vi "SR830-ENBW-WaitTime-Tau-FilterSlope.vi"(8 "error in (no error)":errorcluster, 11 "VISA resource name":refnum<visa-resource-name>) -> (0 "error out":errorcluster, 3 "VISA resource name out":refnum<visa-resource-name>, 4 "Wait Time (s)":dbl, 5 "Filter slope (dB/oct)":dbl, 6 "ENBW":dbl, 7 "Time Constant (s)":dbl)   [LabVIEW 2016]
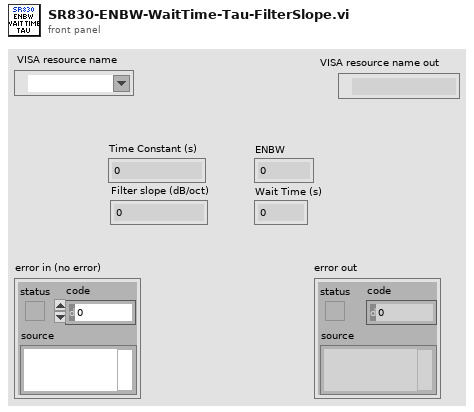
[diagram p1: front panel]
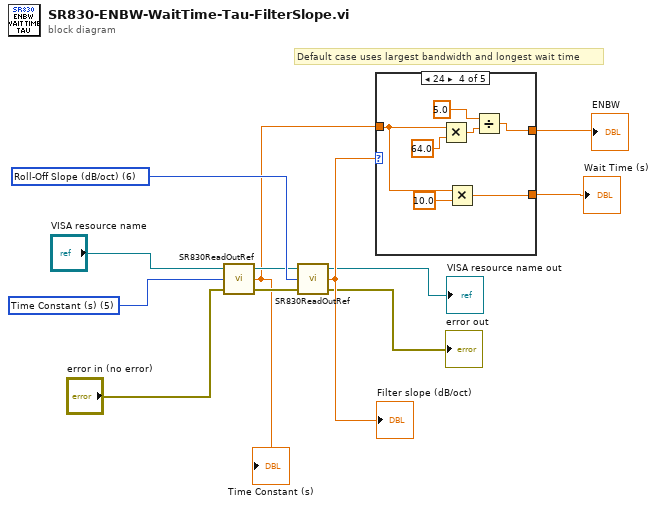
[diagram p0: block diagram]
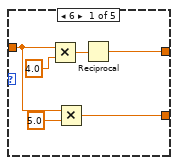
[diagram p2: hidden frame]
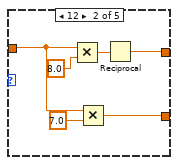
[diagram p3: hidden frame]
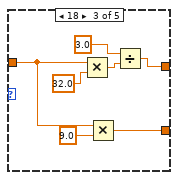
[diagram p4: hidden frame]
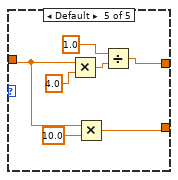
[diagram p5: hidden frame]
diagram:
  w9 = u16 6 items=["Voltage Out (Vrms)"=1, "Frequency (Hz)"=2, "Aux Out 1 (VDC)"=3, "Aux Out 2 (VDC)"=4, "Time Constant (s)"=5, "Roll-Off Slope (dB/oct)"=6] ("ReadOut (1: Voltage Amplitude)")
  w10 = u16 5 items=["Voltage Out (Vrms)"=1, "Frequency (Hz)"=2, "Aux Out 1 (VDC)"=3, "Aux Out 2 (VDC)"=4, "Time Constant (s)"=5, "Roll-Off Slope (dB/oct)"=6] ("ReadOut (1: Voltage Amplitude)")
  # "Default case uses largest bandwidth and longest wait time"
  n1 = call "SR830ReadOutRef.vi"("error in (no error)"="error in (no error)", "ReadOut (1: Voltage Amplitude)"=w10, "VISA resource name"="VISA resource name") -> ("error out"=w8:errorcluster, "ReadOut"=w5:dbl, "VISA resource name out"=w7:refnum<visa-resource-name>)
  "Time Constant (s)" <- w5
  n2 = call "SR830ReadOutRef.vi"("error in (no error)"=w8, "ReadOut (1: Voltage Amplitude)"=w9, "VISA resource name"=w7) -> ("error out"=→"error out":errorcluster, "ReadOut"=w6:dbl, "VISA resource name out"=→"VISA resource name out":refnum<visa-resource-name>)
  "Filter slope (dB/oct)" <- w6
  n3 = case shown="24" w6 {
    tunnel: w5 -> [w15 w21 w28 w32 w39]
    tunnel: [w16 w20 w25 w34 w41] -> w4
    tunnel: [w13 w19 w29 w33 w40] -> w3
    frame 6 {
      n4 = Multiply(x=w15, y=4.0) -> (x*y=w17:dbl)
      n5 = Multiply(x=w15, y=5.0) -> (x*y=w13:dbl)
      n6 = Reciprocal(x=w17) -> (1/x=w16:dbl)
    }
    frame 12 {
      n7 = Multiply(x=w21, y=8.0) -> (x*y=w23:dbl)
      n8 = Multiply(x=w21, y=7.0) -> (x*y=w19:dbl)
      n9 = Reciprocal(x=w23) -> (1/x=w20:dbl)
    }
    frame 18 {
      n10 = Multiply(x=w28, y=32.0) -> (x*y=w27:dbl)
      n11 = Multiply(x=w28, y=9.0) -> (x*y=w29:dbl)
      n12 = Divide(x=3.0, y=w27) -> (x/y=w25:dbl)
    }
    frame 24 {
      n13 = Multiply(x=w32, y=64.0) -> (x*y=w36:dbl)
      n14 = Multiply(x=w32, y=10.0) -> (x*y=w33:dbl)
      n15 = Divide(x=5.0, y=w36) -> (x/y=w34:dbl)
    }
    frame Default {
      n16 = Multiply(x=w39, y=4.0) -> (x*y=w43:dbl)
      n17 = Multiply(x=w39, y=10.0) -> (x*y=w40:dbl)
      n18 = Divide(x=1.0, y=w43) -> (x/y=w41:dbl)
    }
  }
  "ENBW" <- w4
  "Wait Time (s)" <- w3
